vi "TIME_DOWNLOAD.vi"(8 "error in (no error)":errorcluster, 9 "Year,Month,Day,hour,Minute":i64[][](array[numeric]), 10 "appended array":refnum<vi>[](array[refnum])) -> (0 "error out":errorcluster)   [LabVIEW 2017]
panel:
  out "DAY 4":timestamp
  out "DAY 3":timestamp
  out "DAY 2":timestamp
  in  "DAY 1":timestamp format="%<%X\n%x>T"
  out "DAY 1":timestamp
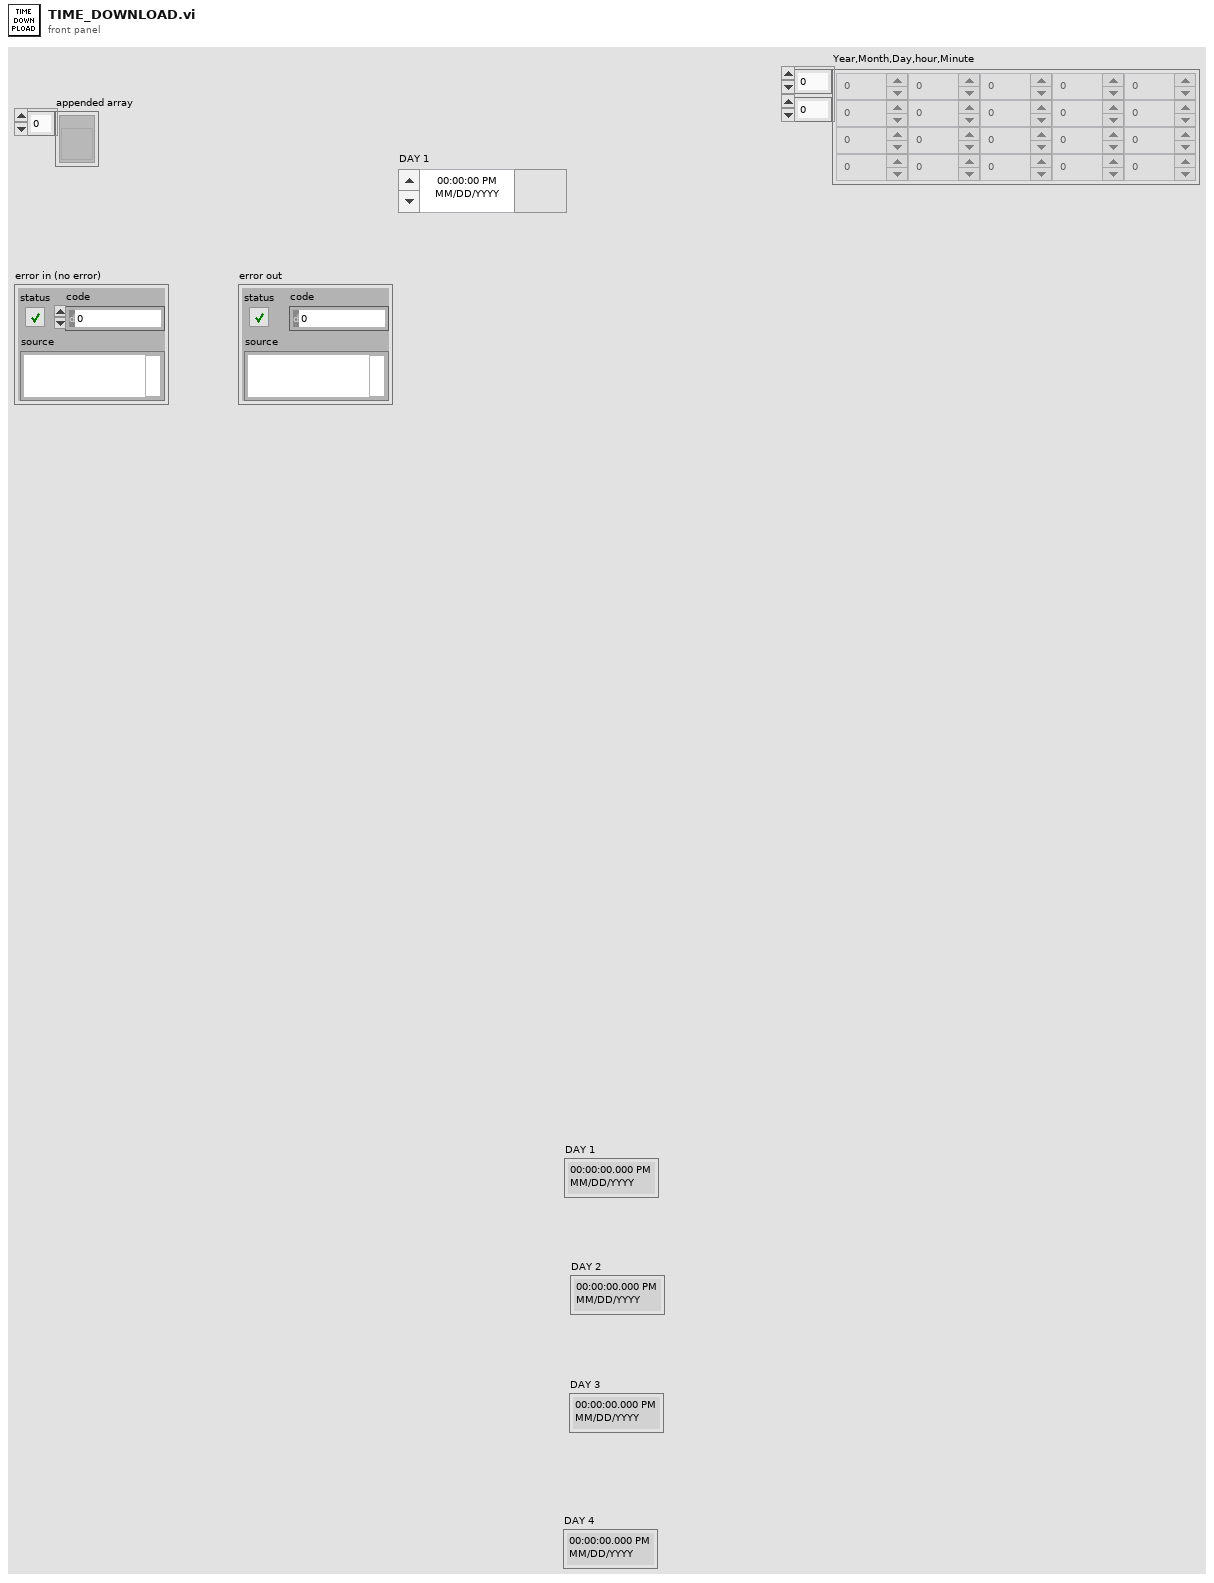
[diagram p1: front panel]
types:
  T1 = cluster{"second":i32, "minute":i32, "hour":i32, "day of month":i32, "month":i32, "year":i32, "day of week":i32, "day of year":i32, "is DST":i32}
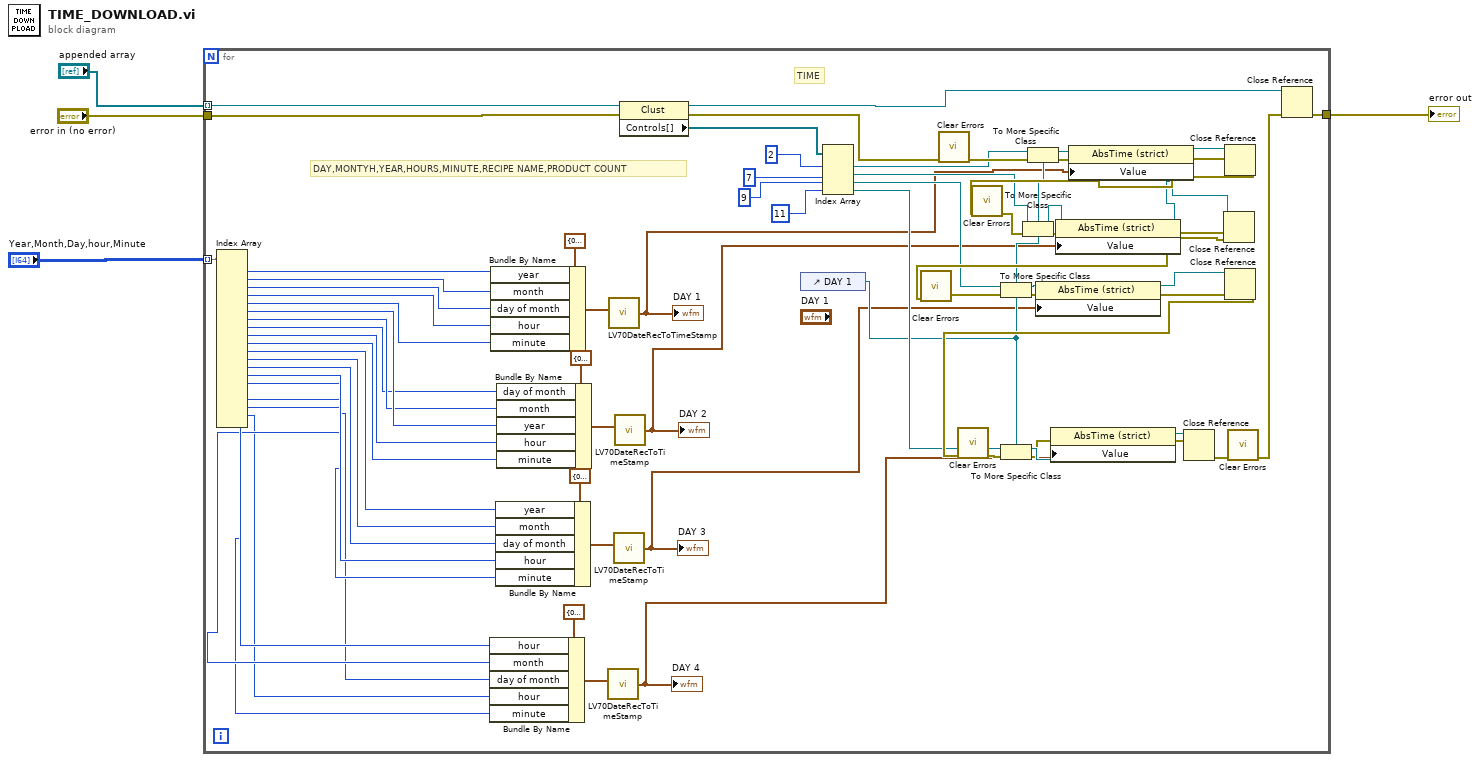
[diagram p0: block diagram]
diagram:
  n1 = for {
    tunnel: [w74] -> w2
    tunnel: "appended array" -> [w77] mode=indexing
    tunnel: "error in (no error)" -> [w76]
    tunnel: "Year,Month,Day,hour,Minute" -> [w44] mode=indexing
    # "DAY,MONTYH,YEAR,HOURS,MINUTE,RECIPE NAME,PRODUCT COUNT"
    # "TIME"
    n2 = Index Array(array=w44) -> (element #1=w8:i64, element #2=w36:i64, element #3=w7:i64, element #4=w35:i64, element #5=w24:i64, element #6=w23:i64, element #7=w22:i64, element #8=w21:i64, element #9=w20:i64, element #10=w19:i64, element #11=w18:i64, element #12=w17:i64, element #13=w16:i64, element #14=w15:i64, element #15=w14:i64, element #16=w13:i64, element #17=w12:i64, element #18=w11:i64, element #19=w10:i64, element #20=w9:i64)  [unwired: 20 in]
    n3 = Bundle By Name(cluster=T1 {"second"=0, "minute"=0, "hour"=0, "day of month"=1, "month"=1, "year"=2018, "day of week"=0, "day of year"=0, "is DST"=0} ("date time rec"), "hour"=w13, "month"=w12, "day of month"=w11, "hour"=w10, "minute"=w9) -> (w29:T1)
    n4 = Bundle By Name(cluster=T1 {"second"=0, "minute"=0, "hour"=0, "day of month"=1, "month"=1, "year"=2018, "day of week"=0, "day of year"=0, "is DST"=0} ("date time rec"), "year"=w8, "month"=w36, "day of month"=w7, "hour"=w35, "minute"=w24) -> (w43:T1)
    n5 = Bundle By Name(cluster=T1 {"second"=0, "minute"=0, "hour"=0, "day of month"=1, "month"=1, "year"=2018, "day of week"=0, "day of year"=0, "is DST"=0} ("date time rec"), "year"=w18, "month"=w17, "day of month"=w16, "hour"=w15, "minute"=w14) -> (w32:T1)
    n6 = Bundle By Name(cluster=T1 {"second"=0, "minute"=0, "hour"=0, "day of month"=1, "month"=1, "year"=2018, "day of week"=0, "day of year"=0, "is DST"=0} ("date time rec"), "day of month"=w21, "month"=w22, "year"=w23, "hour"=w20, "minute"=w19) -> (w33:T1)
    n7 = call <vilib>:"LV70DateRecToTimeStamp.vi"("date time rec"=w29) -> ("Time Stamp"=w26:timestamp)
    "DAY 4" <- w26
    n8 = call <vilib>:"LV70DateRecToTimeStamp.vi"("date time rec"=w43) -> ("Time Stamp"=w37:timestamp)
    "DAY 1" <- w37
    n9 = call <vilib>:"LV70DateRecToTimeStamp.vi"("date time rec"=w32) -> ("Time Stamp"=w27:timestamp)
    "DAY 3" <- w27
    n10 = call <vilib>:"LV70DateRecToTimeStamp.vi"("date time rec"=w33) -> ("Time Stamp"=w28:timestamp)
    "DAY 2" <- w28
    n11 = property class="Clust"(reference=w77, error in=w76) -> (reference out=w73:refnum<vi>, error out=w75:errorcluster, "Controls[]"=w71:refnum<vi>[])
    n12 = control-ref of="DAY 1"() -> (w38:refnum<vi>)
    n13 = Index Array(array=w71, index #1=2 ("index"), index #2=7 ("index"), index #3=9 ("index"), index #4=11 ("index")) -> (element #1=w45:refnum<vi>, element #2=w49:refnum<vi>, element #3=w54:refnum<vi>, element #4=w61:refnum<vi>)
    n14 = call <vilib>:"Clear Errors.vi"("error in (no error)"=w75) -> ("error out"=w48:errorcluster)  [unwired: 5 in, 1 out]
    n15 = To More Specific Class(target class=w38, reference=w45, error in=w48) -> (specific class reference=w46:refnum<vi>, error out=w47:errorcluster)
    n16 = property class="AbsTime (strict)"(reference=w46, error in=w47, "Value"=w37) -> (reference out=w64:refnum<vi>, error out=w72:errorcluster)
    n17 = Close Reference(reference=w64, error in (no error)=w72) -> (error out=w67:errorcluster)
    n18 = call <vilib>:"Clear Errors.vi"("error in (no error)"=w67) -> ("error out"=w52:errorcluster)  [unwired: 5 in, 1 out]
    n19 = To More Specific Class(target class=w38, reference=w49, error in=w52) -> (specific class reference=w50:refnum<vi>, error out=w51:errorcluster)
    n20 = property class="AbsTime (strict)"(reference=w50, error in=w51, "Value"=w28) -> (reference out=w63:refnum<vi>, error out=w69:errorcluster)
    n21 = Close Reference(reference=w63, error in (no error)=w69) -> (error out=w66:errorcluster)
    n22 = call <vilib>:"Clear Errors.vi"("error in (no error)"=w66) -> ("error out"=w55:errorcluster)  [unwired: 5 in, 1 out]
    n23 = To More Specific Class(target class=w38, reference=w54, error in=w55) -> (specific class reference=w53:refnum<vi>, error out=w56:errorcluster)
    n24 = property class="AbsTime (strict)"(reference=w53, error in=w56, "Value"=w27) -> (reference out=w62:refnum<vi>, error out=w68:errorcluster)
    n25 = Close Reference(reference=w62, error in (no error)=w68) -> (error out=w65:errorcluster)
    n26 = call <vilib>:"Clear Errors.vi"("error in (no error)"=w65) -> ("error out"=w58:errorcluster)  [unwired: 5 in, 1 out]
    n27 = To More Specific Class(target class=w38, reference=w61, error in=w58) -> (specific class reference=w59:refnum<vi>, error out=w57:errorcluster)
    n28 = property on="Property Node" class="AbsTime (strict)"(reference=w59, error in=w57, "Value"=w26) -> (reference out=w60:refnum<vi>, error out=w25:errorcluster)
    n29 = Close Reference(reference=w60, error in (no error)=w25) -> (error out=w6:errorcluster)
    n30 = call <vilib>:"Clear Errors.vi"("error in (no error)"=w6) -> ("error out"=w5:errorcluster)  [unwired: 5 in, 1 out]
    n31 = Close Reference(reference=w73, error in (no error)=w5) -> (error out=w74:errorcluster)
  }
  "error out" <- w2
